vi "startedge_red.vi"(1 "4-bit pixmap入力":u8[](array[numeric])) -> (0 "4-bit pixmap出力":u8[](array[numeric]))   [LabVIEW 2016]
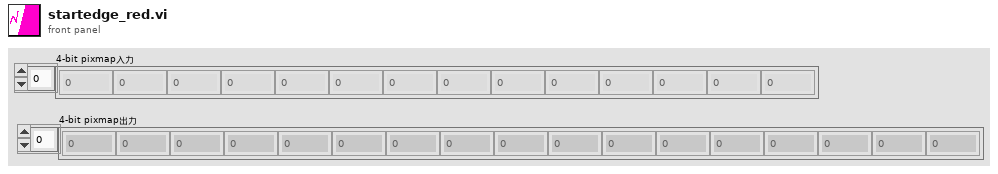
[diagram p1: front panel]
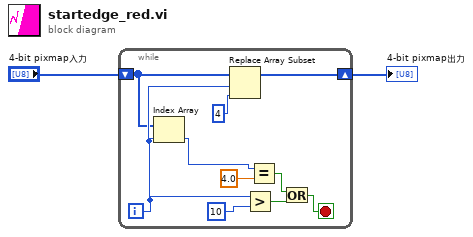
[diagram p0: block diagram]
diagram:
  n1 = while {
    shift-right: [w3] -> w2
    shift-left: "4-bit pixmap入力" -> [w4]
    i -> [w5]
    stop <- w12 stop-if-true
    n2 = Index Array(array=w4, index=w5) -> (element=w7:u8)
    n3 = Replace Array Subset(array=w4, new element=u32 4 ("y"), index=w5) -> (w3:u8[])
    n4 = Greater?(x=w5, y=10) -> (0:w11:bool)
    n5 = Equal?(x=w7, y=4.0) -> (x = y?=w9:bool)
    n6 = Or(x=w9, y=w11) -> (x .or. y?=w12:bool)
  }
  "4-bit pixmap出力" <- w2
